vi "Get Oversample Factor.vi"(0 "Register Buses":T1[](array[typedef]), 11 "error in":errorcluster) -> (4 "Register Buses (out)":T1[](array[typedef]), 6 "sync.meas.oversample factor":u16[](array[numeric]), 15 "error out":errorcluster)   [LabVIEW 2014, in "ni579x Synchronization v2 Host.lvlib"]
doc: "Take a single measurement. It's possible that not all the devices will complete this sucessfully, so make sure the output Measurement Valid is true before using the measurement values."
uses:
  <instrlib>/ni579x/Synchronization/v2/Host/ni579x Synchronization v2 Host.lvlib
  <instrlib>/_niInstr/Register Bus/v0/Host/Public/Register Bus Session.ctl
  <instrlib>/_niInstr/Register Bus/v0/Host/Private/Session Data.ctl
  <instrlib>/ni579x/Synchronization/v2/Shared/ni579x Synchronization Register Addresses.ctl
  <instrlib>/ni579x/Config/v2/Shared/Types/ni579x Register Bus Subsystem ID.ctl
  <instrlib>/_niInstr/Register Bus/v0/Host/Public/Register Read Request.ctl
  <vilib>/Utility/error.llb/Error Cluster From Error Code.vi
  <vilib>/ErrorRing/Error Ring.xnode
  <instrlib>/ni579x/Config/v2/Shared/ni579x Config v2 Shared.lvlib
  <instrlib>/_niInstr/Register Bus/v0/Host/niInstr Register Bus v0 Host.lvlib
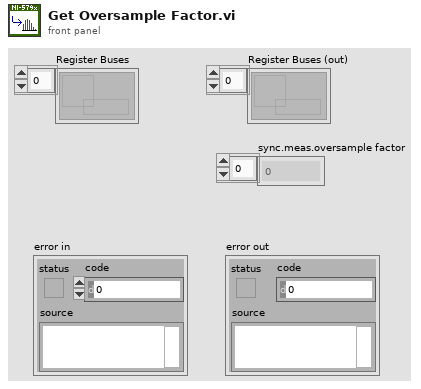
[diagram p1: front panel]
types:
  T1 = typedef "niInstr Register Bus v0 Host.lvlib/Register Bus Session.ctl" = refnum<queue>
  T2 = typedef "niInstr Register Bus v0 Host.lvlib/Register Read Request.ctl" = cluster{"subsystem":u8, "address":u16}
  T3 = typedef "ni579x Config v2 Shared.lvlib/ni579x Register Bus Subsystem ID.ctl" = u8
  T4 = typedef "ni579x Synchronization Register Addresses.ctl" = enum16{"Signature", "Current Version", "Oldest Compatible Version", "Scratch Register", "sync.master", "sync.meas.enable", "sync.meas.ready", "sync.meas.arm", "sync.meas.valid", "sync.meas.value", "sync.cptr.adjust", "sync.cptr.period", "sync.meas.oversample factor"}
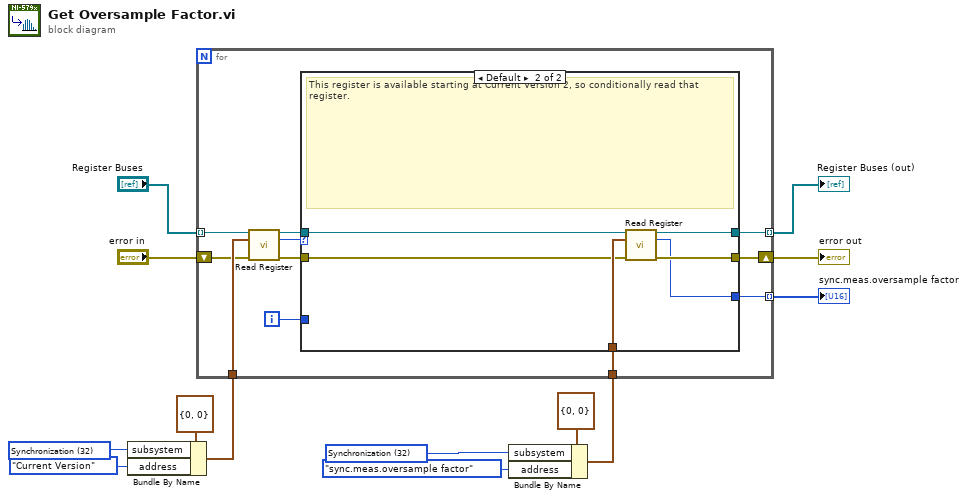
[diagram p0: block diagram]
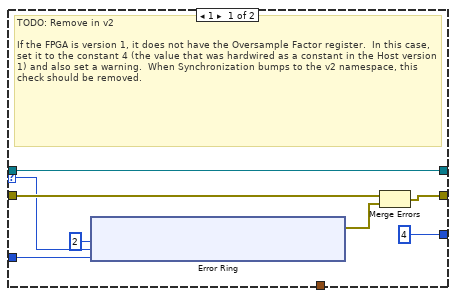
[diagram p2: hidden frame]
diagram:
  w4 = T3 32 items=["FAM Register Operation"=0, "User Command"=16, "Synchronization"=32] ("Subsystem ID")
  w10 = T3 32 items=["FAM Register Operation"=0, "User Command"=16, "Synchronization"=32] ("Subsystem ID")
  n1 = Bundle By Name(cluster=T2 {"subsystem"=0, "address"=0} ("register read request"), "subsystem"=w4, "address"=ni579x_Synchronization_Register_Addresses."Current Version" ("Synchronization Registers")) -> (w3:T2)
  n2 = Bundle By Name(cluster=T2 {"subsystem"=0, "address"=0} ("register read request"), "subsystem"=w10, "address"=ni579x_Synchronization_Register_Addresses."sync.meas.oversample factor" ("Synchronization Registers")) -> (w9:T2)
  n3 = for {
    tunnel: "Register Buses" -> [w19] mode=indexing
    tunnel: [w23] -> w7 mode=indexing
    shift-right: [w24] -> w8
    shift-left: "error in" -> [w18]
    tunnel: w9 -> [w22]
    tunnel: [w21] -> w6 mode=indexing
    tunnel: w3 -> [w20]
    i -> [w14]
    n4 = call <instrlib>:"Read Register.vi"("session in"=w19, "register read request"=w20, "error in"=w18) -> ("session out"=w16:T1, "data"=w15:u32, "error out"=w17:errorcluster)  [unwired: 10 in]
    n5 = case shown="Default" w15 {
      selector: w15 -> [w29 _]
      tunnel: [w30 w47] -> w24
      tunnel: [w26 w46] -> w23
      tunnel: w22 -> [_ w45]
      tunnel: [u32 4 ("data") w44] -> w21
      tunnel: w17 -> [w31 w43]
      tunnel: w16 -> [w26 w42]
      tunnel: w14 -> [w27 _]
      frame 1 {
        # "TODO: Remove in v2\n\nIf the FPGA is version 1, it does not have the Oversample Factor register.  In this case, set it to the constant 4 (the value that was hardwired as a constant in the Host version 1) and also set a warning.  When Synchronization bumps to the v2 namespace, this check should be removed."
        n6 = xnode ("Error Ring")("parameter 0"=2, "parameter 1"=w29, "parameter 2"=w27) -> ("error out"=w32:errorcluster)
        n7 = Merge Errors(w31, w32) -> (w30:errorcluster)
      }
      frame Default {
        # "This register is available starting at Current Version 2, so conditionally read that register."
        n8 = call <instrlib>:"Read Register.vi"("session in"=w42, "register read request"=w45, "error in"=w43) -> ("session out"=w46:T1, "data"=w44:u32, "error out"=w47:errorcluster)  [unwired: 10 in]
      }
    }
  }
  "error out" <- w8
  "Register Buses (out)" <- w7
  "sync.meas.oversample factor" <- w6
